vi "Intersect Circles.vi"(9 "Circle 2":T1 {"Radius" scale=0.0..10.0}, 11 "Circle 1":T1 {"Radius" scale=0.0..10.0}) -> (1 "Point 2":cluster{dbl, dbl}, 3 "Point 1":cluster{dbl, dbl})   [LabVIEW 2023]
panel:
  out "chord halflen":dbl
  out "chord dist":dbl
  out "center dist":sgl
  out "Circles":cluster{"Points":cluster{dbl, dbl}[]}[](graph)
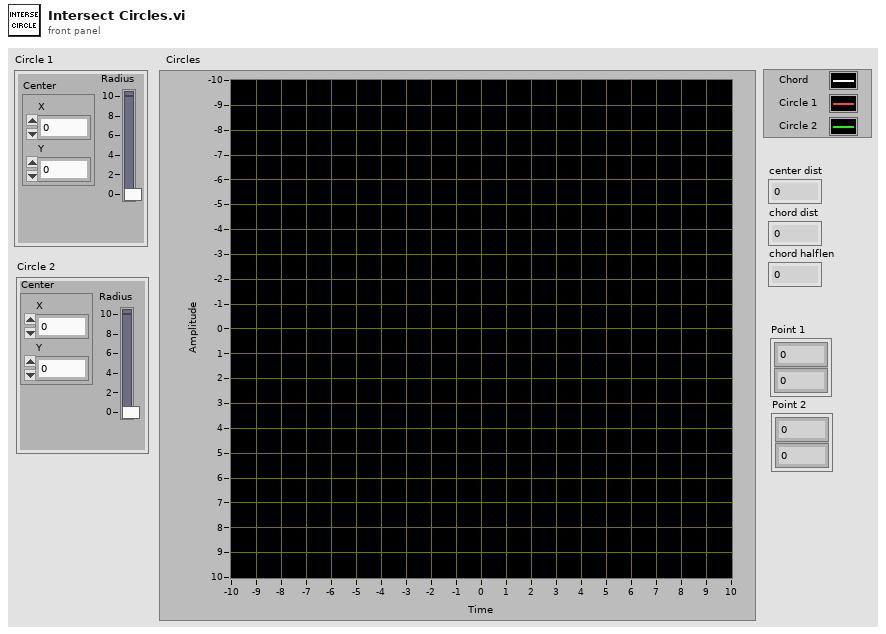
[diagram p1: front panel]
types:
  T1 = cluster{"Center":cluster{"X":sgl, "Y":sgl}, "Radius":dbl}
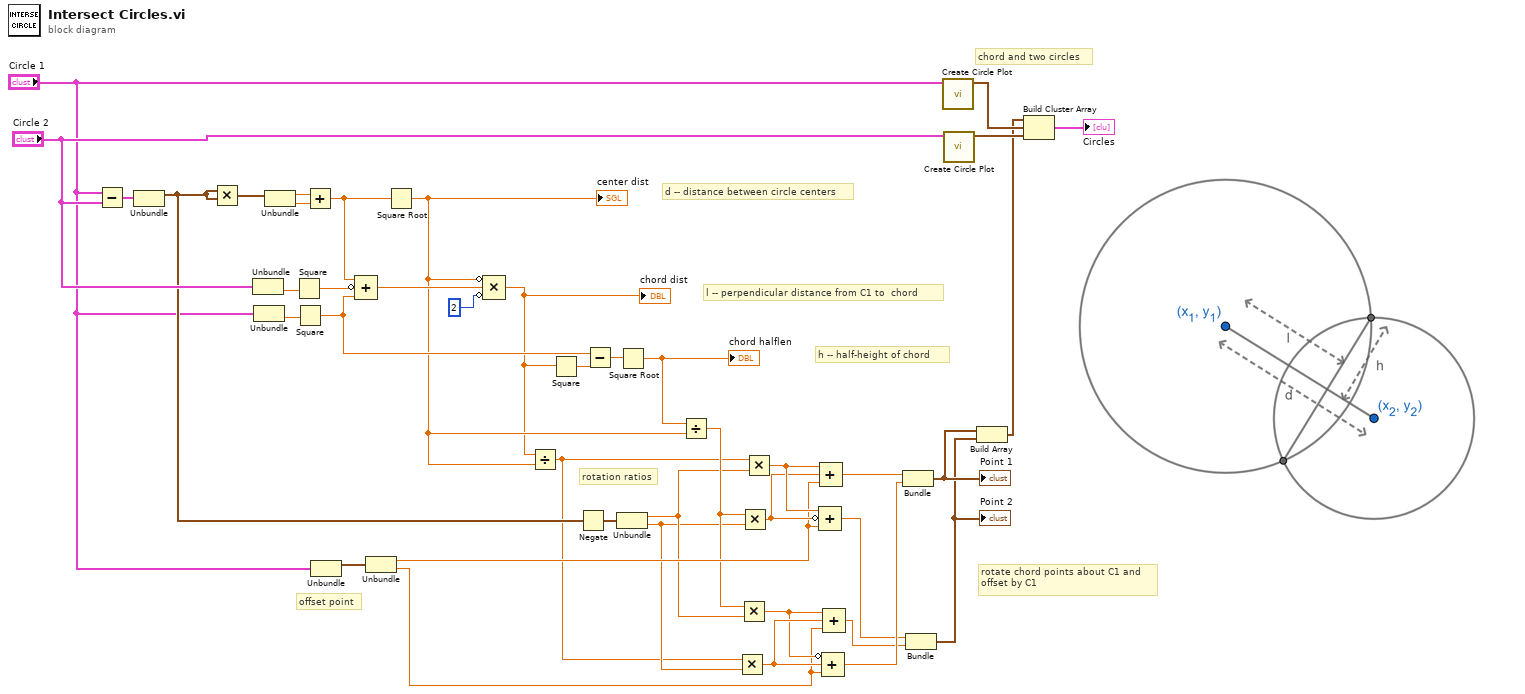
[diagram p0: block diagram]
diagram:
  # "rotation ratios"
  # "offset point"
  # "rotate chord points about C1 and\noffset by C1"
  # "chord and two circles"
  # "h -- half-height of chord"
  # "l -- perpendicular distance from C1 to  chord"
  # "d -- distance between circle centers"
  n1 = Subtract(x="Circle 1", y="Circle 2") -> (x-y=w38:T1)
  n2 = Unbundle(w38) -> ("Center"=w28:cluster{"X":sgl, "Y":sgl})  [unwired: 1 out]
  n3 = Multiply(x=w28, y=w28) -> (x*y=w37:cluster{"X":sgl, "Y":sgl})
  n4 = Unbundle("Circle 2") -> ("Radius"=w33:dbl)  [unwired: 1 out]
  n5 = Unbundle("Circle 1") -> ("Radius"=w34:dbl)  [unwired: 1 out]
  n6 = Unbundle(w37) -> ("X"=w36:sgl, "Y"=w35:sgl)
  n7 = Square(x=w33) -> (x^2=w31:dbl)
  n8 = Square(x=w34) -> (x^2=w7:dbl)
  n9 = Add(x=w36, y=w35) -> (x+y=w11:sgl)
  n10 = Unbundle("Circle 1") -> ("Center"=w24:cluster{"X":sgl, "Y":sgl})  [unwired: 1 out]
  n11 = Compound Arithmetic op=ADD(w11, invert w31, w7) -> (w12:dbl)
  n12 = Unbundle(w24) -> ("X"=w23:sgl, "Y"=w14:sgl)
  n13 = Square Root(x=w11) -> (sqrt(x)=w5:sgl)
  "center dist" <- w5
  n14 = Compound Arithmetic op=MULTIPLY(invert w5, w12, invert 2) -> (w1:dbl)
  "chord dist" <- w1
  n15 = Divide(x=w1, y=w5) -> (x/y=w15:dbl)
  n16 = Square(x=w1) -> (x^2=w30:dbl)
  n17 = Negate(x=w28) -> (-x=w22:cluster{"X":sgl, "Y":sgl})
  n18 = Subtract(x=w7, y=w30) -> (x-y=w29:dbl)
  n19 = Unbundle(w22) -> ("X"=w17:sgl, "Y"=w16:sgl)
  n20 = Square Root(x=w29) -> (sqrt(x)=w21:dbl)
  "chord halflen" <- w21
  n21 = Divide(x=w21, y=w5) -> (x/y=w18:dbl)
  n22 = Multiply(x=w15, y=w16) -> (x*y=w20:dbl)
  n23 = Multiply(x=w18, y=w17) -> (x*y=w19:dbl)
  n24 = Multiply(x=w18, y=w16) -> (x*y=w26:dbl)
  n25 = Multiply(x=w15, y=w17) -> (x*y=w27:dbl)
  n26 = Compound Arithmetic op=ADD(w27, invert w26, w23) -> (w9:dbl)
  n27 = Compound Arithmetic op=ADD(w27, w26, w23) -> (w13:dbl)
  n28 = Compound Arithmetic op=ADD(invert w19, w20, w14) -> (w10:dbl)
  n29 = Compound Arithmetic op=ADD(w19, w20, w14) -> (w8:dbl)
  n30 = Bundle(w13, w10) -> (w4:cluster{dbl, dbl})  [unwired: 1 in]
  "Point 1" <- w4
  n31 = Bundle(w9, w8) -> (w3:cluster{dbl, dbl})  [unwired: 1 in]
  "Point 2" <- w3
  n32 = call "Create Circle Plot.vi"("Circle Descr"="Circle 1") -> ("Points"=w41:cluster{dbl, dbl}[])  [unwired: 10 in]
  n33 = call "Create Circle Plot.vi"("Circle Descr"="Circle 2") -> ("Points"=w40:cluster{dbl, dbl}[])  [unwired: 10 in]
  n34 = Build Array(w4, w3) -> (w2:cluster{dbl, dbl}[])
  n35 = Build Cluster Array(w2, w41, w40) -> (→"Circles":cluster{"Points":cluster{dbl, dbl}[]}[])
